vi "client parse client status.vi"(8 "error in (no error)":errorcluster, 11 "Client IP":string) -> (0 "error out":errorcluster, 1 "Update Needed?":bool, 2 "Client Detected?":bool, 3 "Client Status Keys":T1)   [LabVIEW 2011]
uses:
  ITK EXT/utils/keyedarr.llb/Keyed Array.ctl
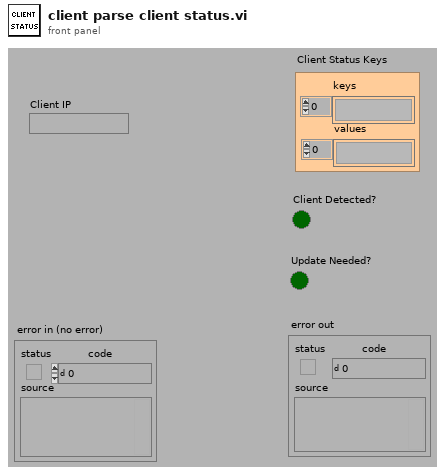
[diagram p1: front panel]
types:
  T1 = typedef "Keyed Array.ctl" = cluster{"keys":string[], "values":string[]}
  T2 = enum16{"Version 1 < Version 2", "Version 1 = Version 2", "Version 1 > Version 2"}
  T3 = typedef "OGAB Version.ctl" = cluster{"Version":string, "Build Number":u32, "Build Date/Time":dbl}
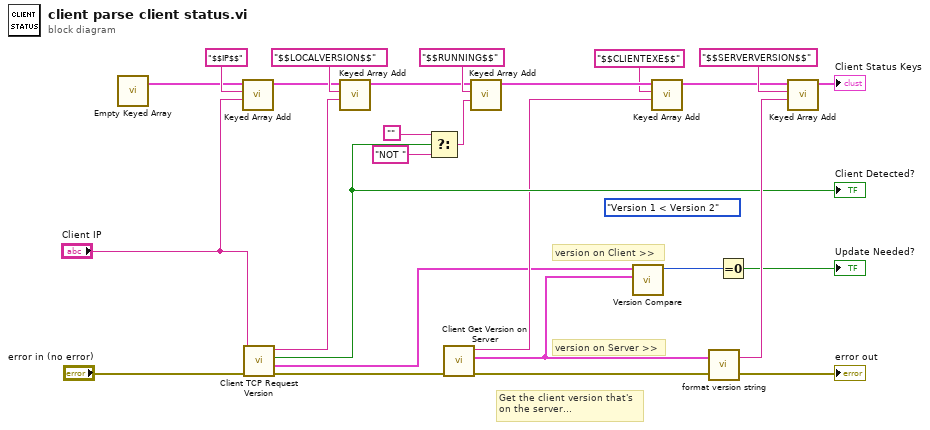
[diagram p0: block diagram]
diagram:
  (unwired) T2."Version 1 < Version 2" ("x")
  # "version on Server >>"
  # "version on Client >>"
  # "Get the client version that's\non the server..."
  n1 = call "Empty Keyed Array.vi"() -> ("empty keyed array"=w20:T1)  [unwired: 3 out]
  n2 = call "Keyed Array Add.vi"("value"="Client IP", "key"="$$IP$$" ("Template (\"\")"), "array in"=w20) -> ("array out"=w15:T1)  [unwired: 1 in, 3 out]
  n3 = call "Client TCP Request Version.vi"("error in (no error)"="error in (no error)", "Client IP"="Client IP") -> ("error out"=w10:errorcluster, "Client Version"=w3:T3, "Client Detected?"=w11:bool, "Client Version String"=w13:string)  [unwired: 6 out]
  "Client Detected?" <- w11
  n4 = call "Keyed Array Add.vi"("value"=w13, "key"="$$LOCALVERSION$$" ("Template (\"\")"), "array in"=w15) -> ("array out"=w12:T1)  [unwired: 1 in, 3 out]
  n5 = Select(t="", s=w11, f="NOT " ("Template (\"\")")) -> (s? t:f=w17:string)
  n6 = call "Client Get Version on Server.vi"("error in (no error)"=w10) -> ("error out"=→"error out":errorcluster, "Version"=w2:T3, "Client EXE Name"=w5:string)  [unwired: 8 out]
  n7 = call "Keyed Array Add.vi"("value"=w17, "key"="$$RUNNING$$" ("Template (\"\")"), "array in"=w12) -> ("array out"=w8:T1)  [unwired: 1 in, 3 out]
  n8 = call "Version Compare.vi"("Version 1"=w3, "Version 2"=w2) -> ("Version Comparison"=w4:T2)  [unwired: 1 in, 5 out]
  n9 = call "Keyed Array Add.vi"("value"=w5, "key"="$$CLIENTEXE$$" ("Template (\"\")"), "array in"=w8) -> ("array out"=w7:T1)  [unwired: 1 in, 3 out]
  n10 = call "format version string.vi"("Version"=w2) -> ("Version String"=w19:string)  [unwired: 2 out]
  n11 = Equal To 0?(x=w4) -> (x = 0?=→"Update Needed?":bool)
  n12 = call "Keyed Array Add.vi"("value"=w19, "key"="$$SERVERVERSION$$" ("Template (\"\")"), "array in"=w7) -> ("array out"=→"Client Status Keys":T1)  [unwired: 1 in, 3 out]
